vi "STFT Spectrograms (obs 85).vi"(9 "window info":cluster{"type":u32, "length":i32}={"type"=0, "length"=64} {"type" items=["Rectangle"=0, "Hanning"=1, "Hamming"=2, "Blackman-Harris"=3, "Exact Blackman"=4, "Blackman"=5, "Flat Top"=6, "4 Term B-Harris "=7, "7 Term B-Harris"=8, "Low Sidelobe"=9, "Blackman Nuttall"=11, "Triangle"=30, "Gaussian"=62]}, 10 "time-freq sampling info":cluster{"time steps":i32, "frequency bins":i32}={"time steps"=-1, "frequency bins"=512}, 11 "X":dbl[](array[numeric])) -> (0 "error":i32, 3 "STFT Spectrogram {X}":dbl[][](array[numeric]))   [LabVIEW 2017, in "NI_Gmath.lvlib"]
doc: "The STFT Spectrograms VI was rewritten with two new inputs in LabVIEW 8.6. Replace this VI with an STFT Spectrograms VI from the <B>Functions</B> palette to use the new functionality. \n\nComputes the signal energy distribution in the joint time-frequency domain, using the short-time Fourier transform (STFT) algorithm. The STFT Spectrograms VI performs a sliding FFT.\n\nTo compute <B>STFT Spectrogram {X}</B>, this VI first computes the STFT of <B>X</B>. To compute the STFT of <B>X</B>, this VI uses a sliding window to divide the signal into several blocks of data. The VI then applies an N-points fast Fourier transform to each block of data to obtain the frequency contents of each block of data, where N is <B>frequency bins</B>. The STFT aligns the center of the first sliding window with the first sample of the signal <B>X</B> and extends the beginning of the signal by adding zeros. The sliding window moves <B>time steps</B> samples to the next block of data. If the window moves out of <B>X</B>, this VI pads <B>X</B> with zeros."
uses:
  <vilib>/gmath/NI_Gmath.lvlib
  <vilib>/Analysis/baseanly.llb/Unit Vector (DBL).vi
  <vilib>/Analysis/2dsp.llb/Real FFT.vi
  <vilib>/Analysis/0measdsp.llb/Scaled Time Domain Window (DBL).vi
  <vilib>/Analysis/NI_AALPro.lvlib
  <vilib>/Analysis/NI_AALBase.lvlib
panel:
  # "This VI is obsolete !!!\nYou should replace this VI in your diagram with the STFT Spectrograms VI."
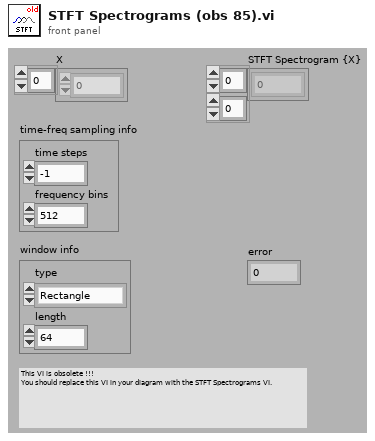
[diagram p1: front panel]
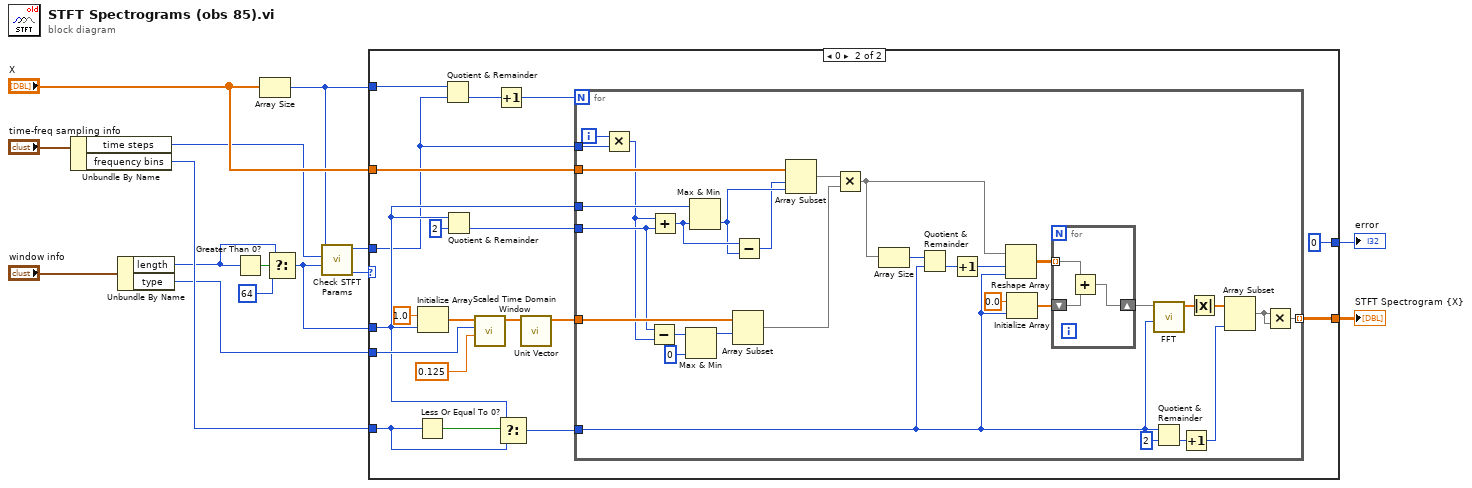
[diagram p0: block diagram]
diagram:
  n1 = Unbundle By Name("time-freq sampling info") -> ("time steps"=w6:i32, "frequency bins"=w5:i32)
  n2 = Unbundle By Name("window info") -> ("length"=w3:i32, "type"=w2:u32)
  n3 = Greater Than 0?(x=w3) -> (x > 0?=w10:bool)
  n4 = Array Size(array="X") -> (size(s)=w13:i32)
  n5 = Select(t=w3, s=w10, f=64) -> (s? t:f=w8:i32)
  n6 = call <vilib>:"Check STFT Params.vi"("windows length"=w8, "time increment"=w6, "len(X)"=w13) -> ("error"=w12:i32, "time step out"=w1:i32)  [unwired: 1 in, 6 out]
  n7 = case shown="0" w12 {
    selector: w12 -> [w16 _]
    tunnel: w2 -> [_ w24]
    tunnel: "X" -> [_ w29]
    tunnel: w8 -> [_ w21]
    tunnel: w5 -> [_ w22]
    tunnel: [_ w32] -> w15
    tunnel: w13 -> [_ w26]
    tunnel: [w16 0] -> w11
    tunnel: w1 -> [_ w17]
    frame Default {
    }
    frame 0 {
      n8 = Less Or Equal To 0?(x=w22) -> (x <= 0?=w28:bool)
      n9 = Initialize Array(1.0 ("element"), w21) -> (w25:dbl[])
      n10 = Quotient & Remainder(x=w26, y=w17) -> (floor(x/y)=w31:i32)  [unwired: 1 out]
      n11 = Quotient & Remainder(x=w21, y=2) -> (floor(x/y)=w33:i32)  [unwired: 1 out]
      n12 = call-poly <vilib>:"Scaled Time Domain Window.vi"("window parameter"=0.125, "window"=w24, "X"=w25) -> ("Windowed X"=w23:dbl[])  [unwired: 8 out]
      n13 = Increment(x=w31) -> (x+1=w20:i32)
      n14 = Select(t=w21, s=w28, f=w22) -> (s? t:f=w27:i32)
      n15 = call-poly <vilib>:"Unit Vector.vi"("Input Vector"=w23) -> ("Unit Vector"=w30:dbl[])  [unwired: 2 in, 8 out]
      n16 = for {
        N: w20 -> [_]
        tunnel: w29 -> [w64]
        tunnel: w17 -> [w65]
        tunnel: w33 -> [w59]
        tunnel: w21 -> [w63]
        tunnel: w30 -> [w62]
        tunnel: w27 -> [w41]
        tunnel: [w42] -> w32 mode=indexing
        i -> [w66]
        n17 = Multiply(x=w66, y=w65) -> (x*y=w58:i32)
        n18 = Subtract(x=w59, y=w58) -> (x-y=w57:i32)
        n19 = Add(x=w58, y=w59) -> (x+y=w54:i32)
        n20 = Max & Min(x=w57, y=0) -> (max(x,y)=w55:i32)  [unwired: 1 out]
        n21 = Max & Min(x=w63, y=w54) -> (min(x,y)=w53:i32)  [unwired: 1 out]
        n22 = Array Subset(array=w62, index=w55) -> (w60:dbl[])  [unwired: 1 in]
        n23 = Subtract(x=w54, y=w53) -> (x-y=w52:i32)
        n24 = Array Subset(array=w64, index=w52, length=w53) -> (w61:dbl[])
        n25 = Multiply(x=w61, y=w60) -> (x*y=w50:dbl[])
        n26 = Array Size(array=w50) -> (size(s)=w49:i32)
        n27 = Quotient & Remainder(x=w49, y=w41) -> (floor(x/y)=w37:i32)  [unwired: 1 out]
        n28 = Increment(x=w37) -> (x+1=w36:i32)
        n29 = Reshape Array(w50, w36, w41) -> (w47:dbl[][])
        n30 = Initialize Array(0.0 ("element"), w41) -> (w48:dbl[])
        n31 = for {
          tunnel: w47 -> [w69] mode=indexing
          shift-right: [w67] -> w46
          shift-left: w48 -> [w68]
          n32 = Add(x=w69, y=w68) -> (x+y=w67:dbl[])
        }
        n33 = call-poly <vilib>:"FFT.vi"("FFT size"=w41, "X"=w46) -> ("FFT {X}"=w45:cdb[])  [unwired: 1 in, 8 out]
        n34 = Quotient & Remainder(x=w41, y=2) -> (floor(x/y)=w39:i32)  [unwired: 1 out]
        n35 = Increment(x=w39) -> (x+1=w38:i32)
        n36 = Absolute Value(x=w45) -> (abs(x)=w44:dbl[])
        n37 = Array Subset(array=w44, length=w38) -> (w43:dbl[])  [unwired: 1 in]
        n38 = Multiply(x=w43, y=w43) -> (x*y=w42:dbl[])
      }
    }
  }
  "STFT Spectrogram {X}" <- w15
  "error" <- w11
